vi "Port To Labels.vi"(8 "error in":errorcluster, 11 "port ref":T6 format="%.0x") -> (0 "error out":errorcluster, 2 "labels":T1[](array[typedef]), 3 "port ref out":T6 format="%.0x")   [LabVIEW 2020, in "AIM ARINC 429 Scripting.lvlib"]
uses:
  AIM ARINC 429 Scripting.lvlib
  Shared/Transfer Type.ctl
  <vilib>/NI/NI VeriStand Encoding and Decoding/Encoding.ctl
  <vilib>/NI/NI VeriStand Encoding and Decoding/Encoding and Decoding.lvlib
  Shared/Parameter Definition.ctl
  Shared/VS Channel Definition for Parameter.ctl
  Shared/VS Channels Definition for Label.ctl
  <vilib>/NI VeriStand/Custom Device API/Custom Device Item Ref.ctl
  <vilib>/NI VeriStand/Custom Device API/Custom Device API.lvlib
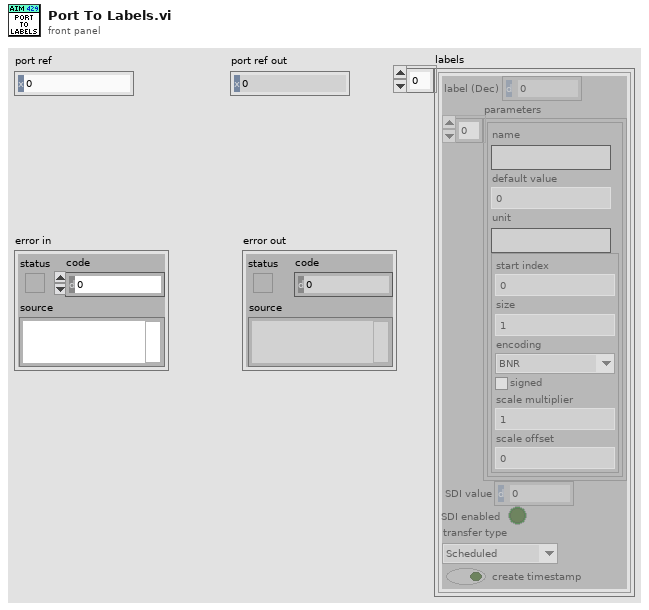
[diagram p1: front panel]
types:
  T1 = typedef "VS Channels Definition for Label.ctl" = cluster{"label (Dec)":u32, "parameters":T2[], "SDI value":u8, "SDI enabled":bool, "transfer type":T5, "create timestamp":bool}
  T2 = typedef "VS Channel Definition for Parameter.ctl" = cluster{"name":string, "default value":dbl, "unit":string, "Parameter":T3}
  T3 = typedef "Parameter Definition.ctl" = cluster{"start index":i32, "size":i32, "encoding":T4, "signed":bool, "scale multiplier":dbl, "scale offset":dbl}
  T4 = typedef "Encoding and Decoding.lvlib/Encoding.ctl" = enum16{"BNR", "BCD", "Discrete"}
  T5 = typedef "Transfer Type.ctl" = enum16{"Scheduled", "Acyclic", "Block", "Strobe"}
  T6 = typedef "Custom Device API.lvlib/Custom Device Item Ref.ctl" = u64
  T7 = typedef "Label Properties.ctl" = cluster{"label (Dec)":T8, "SDI value":u8, "SDI enabled":bool}
  T8 = typedef "Label.ctl" = u8
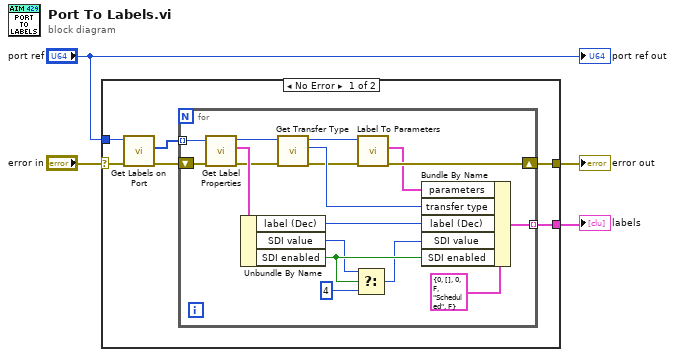
[diagram p0: block diagram]
diagram:
  n1 = case shown="No Error" "error in" {
    selector: "error in" -> [w5 w28]
    tunnel: "port ref" -> [w6 _]
    tunnel: [w9 w28] -> w4
    tunnel: [w10 _] -> w1
    frame No Error {
      n2 = call "Get Labels on Port.vi"("error in"=w5, "port in"=w6) -> ("error out"=w8:errorcluster, "labels"=w7:T6[])  [unwired: 6 in, 2 out]
      n3 = for {
        tunnel: w7 -> [w26] mode=indexing
        tunnel: [w12] -> w10 mode=indexing
        shift-right: [w13] -> w9
        shift-left: w8 -> [w27]
        n4 = call "Get Label Properties.vi"("error in"=w27, "label ref in"=w26) -> ("error out"=w23:errorcluster, "label properties"=w24:T7, "label ref out"=w22:T6)  [unwired: 6 in, 1 out]
        n5 = Unbundle By Name(w24) -> ("label (Dec)"=w20:T8, "SDI value"=w18:u8, "SDI enabled"=w19:bool)
        n6 = call "Get Transfer Type.vi"("error in"=w23, "label ref in"=w22) -> ("error out"=w15:errorcluster, "transfer type"=w21:T5, "label ref out"=w14:T6)  [unwired: 7 in]
        n7 = Select(t=w18, s=w19, f=u8 4 ("SDI value")) -> (s? t:f=w16:u8)
        n8 = call "Label To Parameters.vi"("error in"=w15, "label ref"=w14) -> ("error out"=w13:errorcluster, "parameters"=w11:T2[])  [unwired: 7 in, 1 out]
        n9 = Bundle By Name(cluster=T1 {"label (Dec)"=0, "parameters"=[], "SDI value"=0, "SDI enabled"=FALSE, "transfer type"=enum."Scheduled", "create timestamp"=FALSE} ("label parameters"), "parameters"=w11, "transfer type"=w21, "label (Dec)"=w20, "SDI value"=w16, "SDI enabled"=w19) -> (w12:T1)
      }
    }
    frame Error {
    }
  }
  "error out" <- w4
  "labels" <- w1
  "port ref out" <- "port ref"
